vi "BuildClassInstaller.vi"() -> ()   [LabVIEW 2019]
panel:
  out "error out":errorcluster
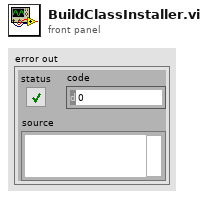
[diagram p1: front panel]
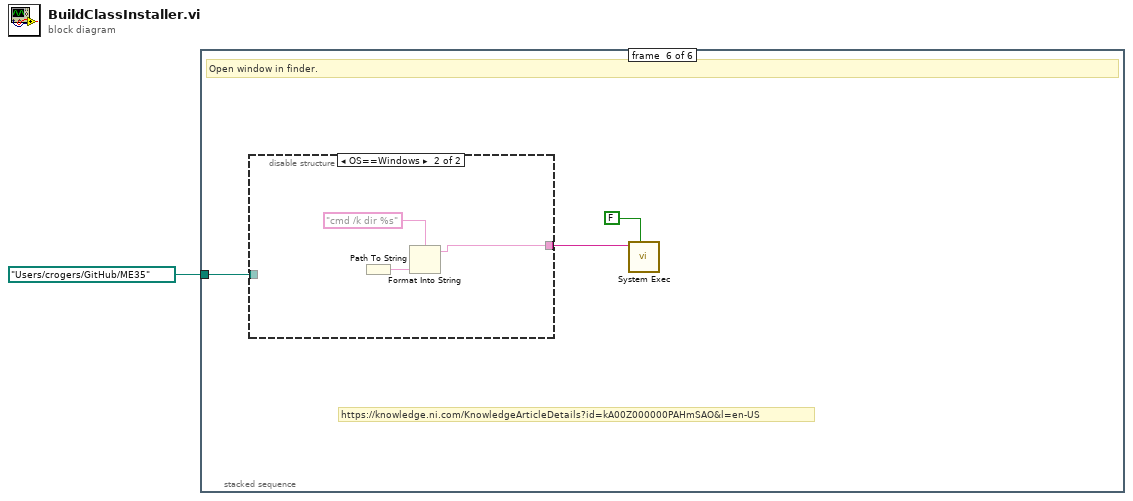
[diagram p0: block diagram]
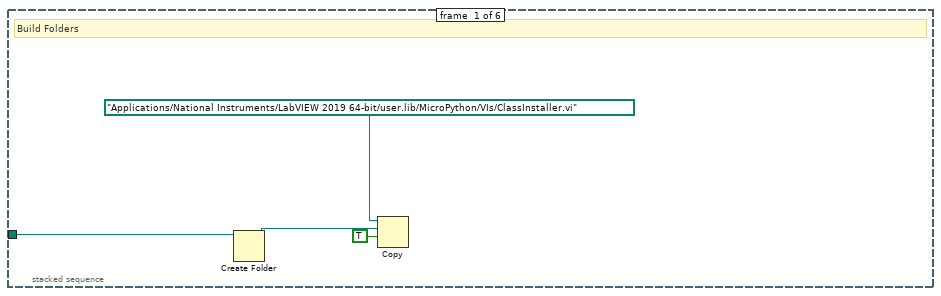
[diagram p2: hidden frame]
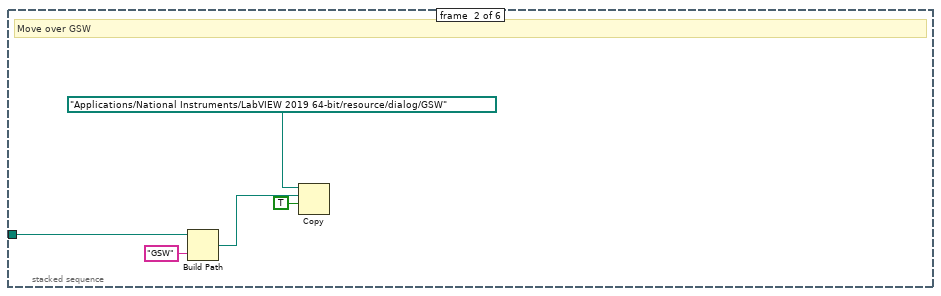
[diagram p3: hidden frame]
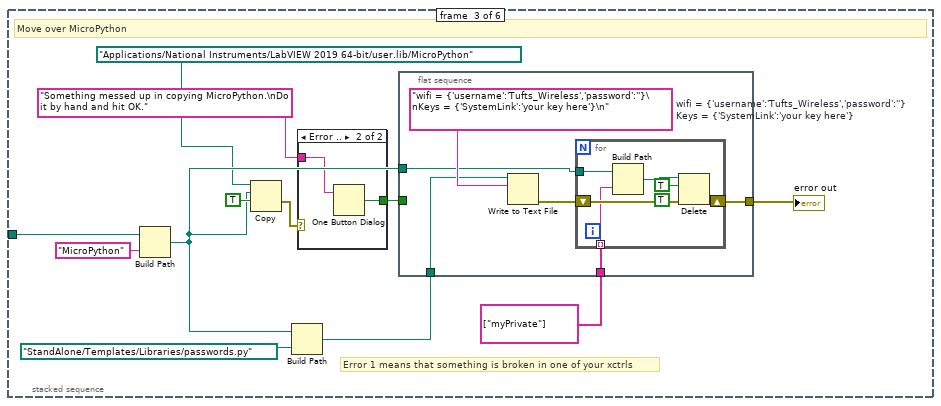
[diagram p4: hidden frame]
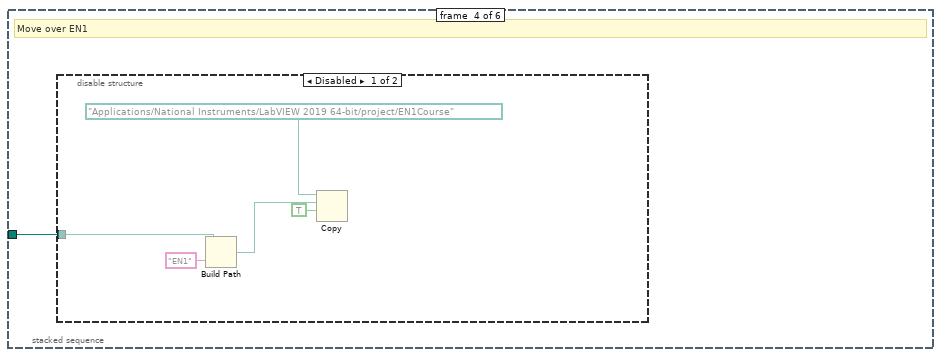
[diagram p6: hidden frame]
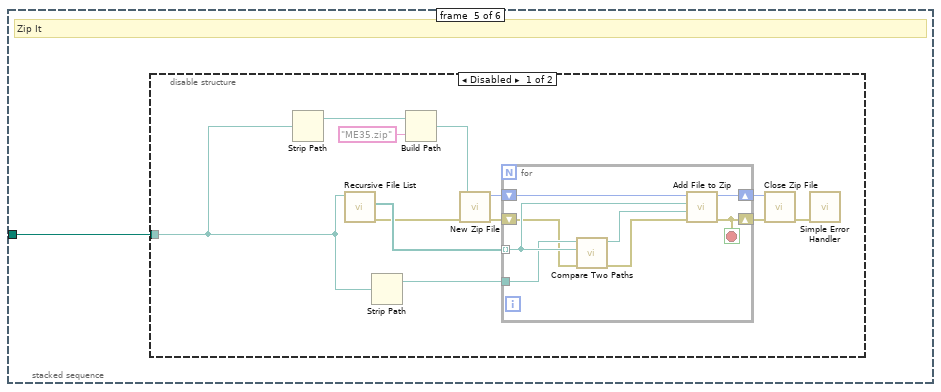
[diagram p8: hidden frame]
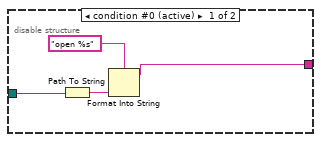
[diagram p10: hidden frame]
diagram:
  n1 = stacked-sequence {
    tunnel: path "/Users/crogers/GitHub/ME35" ("Path") -> [w5 w7 w17 w38 w44 w67]
    frame #0 {
      # "Build Folders"
      n2 = Create Folder(path (use dialog)=w5) -> (created path=w3:path)  [unwired: 2 in, 2 out]
      n3 = Copy(9:TRUE ("overwrite (F)"), 10:w3, 11:path "/Applications/National Instruments/LabVIEW 2019 64-bit/user.lib/MicroPython/VIs/ClassInstaller.vi" ("Path")) -> ()  [unwired: 2 in, 3 out]
    }
    frame #1 {
      # "Move over GSW"
      n4 = Build Path(base path=w7, name or relative path="GSW") -> (appended path=w8:path)
      n5 = Copy(9:TRUE ("overwrite (F)"), 10:w8, 11:path "/Applications/National Instruments/LabVIEW 2019 64-bit/resource/dialog/GSW" ("Path")) -> ()  [unwired: 2 in, 3 out]
    }
    frame #2 {
      # "Error 1 means that something is broken in one of your xctrls"
      # "Move over MicroPython"
      n6 = Build Path(base path=w17, name or relative path="MicroPython") -> (appended path=w15:path)
      n7 = Copy(9:TRUE ("overwrite (F)"), 10:w15, 11:path "/Applications/National Instruments/LabVIEW 2019 64-bit/user.lib/MicroPython" ("Path")) -> (0:w13:errorcluster)  [unwired: 2 in, 2 out]
      n8 = Build Path(base path=w15, name or relative path=path "StandAlone/Templates/Libraries/passwords.py" ("Path")) -> (appended path=w21:path)
      n9 = case shown="Error .." w13 {
        tunnel: [_ w24] -> w12
        tunnel: "Something messed up in copying MicroPython.\nDo it by hand and hit OK." ("name or relative path") -> [_ w23]
        frame No Error {
        }
        frame Error {
          n10 = One Button Dialog(message=w23) -> (true=w24:bool)  [unwired: 1 in]
        }
      }
      n11 = flat-sequence {
        tunnel: w21 -> [w29]
        tunnel: string[] ["myPrivate"] -> [w27]
        tunnel: [w26] -> w18
        tunnel: w15 -> [w25]
        tunnel: w12 -> [_]
        frame #0 {
          w30 = "wifi = {'username':'Tufts_Wireless','password':''}\nKeys = {'SystemLink':'your key here'}\n"  # wifi = {'username':'Tufts_Wireless','password':''} Keys = {'SystemLink':'your key here'}
          n12 = Write to Text File(file (use dialog)=w29, text=w30) -> (error out=w28:errorcluster)  [unwired: 2 in, 2 out]
          n13 = for {
            tunnel: w25 -> [w36]
            tunnel: w27 -> [w31] mode=indexing
            shift-right: [w32] -> w26
            shift-left: w28 -> [w37]
            n14 = Build Path(base path=w36, name or relative path=w31) -> (appended path=w35:path)
            n15 = Delete(path (use dialog)=w35, entire hierarchy (F)=TRUE, confirm (F)=TRUE, error in=w37) -> (error out=w32:errorcluster)  [unwired: 1 in, 2 out]
          }
        }
      }
      "error out" <- w18
    }
    frame #3 {
      # "Move over EN1"
      n16 = disable-structure shown="Disabled" {
        disable-tunnel: w38 -> [w40 _]
        frame Disabled {
          n17 = Build Path(base path=w40, name or relative path="EN1") -> (appended path=w41:path)
          n18 = Copy(9:TRUE ("overwrite (F)"), 10:w41, 11:path "/Applications/National Instruments/LabVIEW 2019 64-bit/project/EN1Course" ("Path")) -> ()  [unwired: 2 in, 3 out]
        }
        frame Enabled {
        }
      }
    }
    frame #4 {
      # "Zip It"
      n19 = disable-structure shown="Disabled" {
        disable-tunnel: w44 -> [w48 _]
        frame Disabled {
          n20 = Strip Path(path=w48) -> (stripped path=w47:path)  [unwired: 1 out]
          n21 = call <vilib>:"Recursive File List.vi"("Folder Path"=w48) -> ("error out"=w54:errorcluster, "All Files in Dir"=w55:path[])  [unwired: 6 in, 3 out]
          n22 = Strip Path(path=w48) -> (stripped path=w56:path)  [unwired: 1 out]
          n23 = Build Path(base path=w47, name or relative path="ME35.zip") -> (appended path=w46:path)
          n24 = call <vilib>:"New Zip File.vi"("error in (no error)"=w54, "target"=w46) -> ("error out"=w51:errorcluster, "zip file out"=w50:i64)  [unwired: 1 in, 3 out]
          n25 = for {
            tunnel: w55 -> [w61] mode=indexing
            shift-right: [w63] -> w53
            shift-left: w50 -> [w64]
            tunnel: w56 -> [w60]
            shift-right: [w62] -> w52
            shift-left: w51 -> [w58]
            stop <- w62 stop-if-true
            n26 = call <vilib>:"Compare Two Paths.vi"("error in (no error)"=w58, "Path 2"=w61, "Path 1"=w60) -> ("error out"=w57:errorcluster, "Relative Path from 1 to 2"=w59:path)  [unwired: 5 in, 2 out]
            n27 = call <vilib>:"Add File to Zip.vi"("error in (no error)"=w57, "destination path in zip"=w59, "source file path"=w61, "zip file in"=w64) -> ("error out"=w62:errorcluster, "zip file out"=w63:i64)  [unwired: 6 out]
          }
          n28 = call <vilib>:"Close Zip File.vi"("error in (no error)"=w52, "zip file in"=w53) -> ("error out"=w49:errorcluster)  [unwired: 1 in, 4 out]
          n29 = call <vilib>:"Simple Error Handler.vi"("error in (no error)"=w49) -> ()  [unwired: 1 in, 8 out]
        }
        frame Enabled {
        }
      }
    }
    frame #5 {
      # "https://knowledge.ni.com/KnowledgeArticleDetails?id=kA00Z000000PAHmSAO&l=en-US"
      # "Open window in finder."
      n30 = disable-structure shown="OS==Windows" {
        disable-tunnel: w67 -> [w71 _]
        disable-tunnel: [w68 w72] -> w65
        frame condition #0 (active) {
          n31 = Path To String(path=w71) -> (string=w70:string)
          n32 = Format Into String(format string="open %s", w70) -> (resulting string=w68:string)  [unwired: 2 in, 1 out]
        }
        frame condition #1 {
          n33 = Path To String() -> (string=w74:string)  [unwired: 1 in]
          n34 = Format Into String(format string="cmd /k dir %s", w74) -> (resulting string=w72:string)  [unwired: 2 in, 1 out]
        }
      }
      n35 = call <vilib>:"System Exec.vi"("wait until completion? (T)"=FALSE, "command line"=w65) -> ()  [unwired: 6 in, 4 out]
    }
  }
